vi "plot_parseDisdrometer.vi"(0 "Current Data":dbl[][](array[numeric]), 5 "Yesterday's Data":dbl[][](array[numeric])) -> (4 "Plot 1":T1(array[cluster]), 8 "Plot 2":T2(array[cluster]))   [LabVIEW 2018]
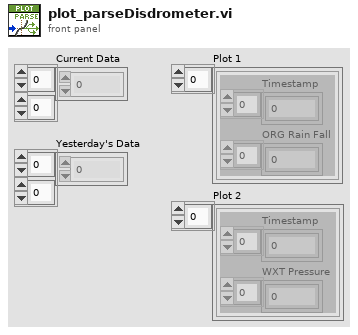
[diagram p1: front panel]
types:
  T1 = cluster{"Timestamp":dbl[], "ORG Rain Fall":dbl[]}[]
  T2 = cluster{"Timestamp":dbl[], "WXT Pressure":dbl[]}[]
  T3 = cluster{"Timestamp":dbl[], "Disdrometer Rain Rate":dbl[]}
  T4 = cluster{"Timestamp":dbl[], "Disdrometer Rain Rate":dbl[], "Disdrometer Rain Fall":dbl[]}
  T5 = cluster{"Timestamp":dbl[], "Disdrometer Rain Fall":dbl[]}
  T6 = cluster{"Timestamp":dbl[], "Disdrometer Rain Rate":dbl[]}[]
  T7 = cluster{"Timestamp":dbl[], "Disdrometer Rain Fall":dbl[]}[]
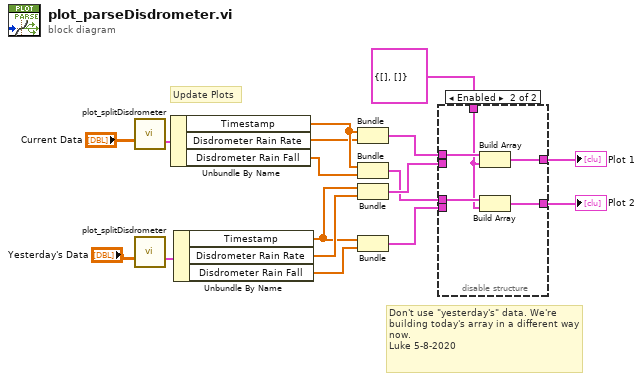
[diagram p0: block diagram]
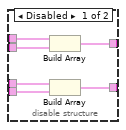
[diagram p2: hidden frame]
diagram:
  # "Don't use \"yesterday's\" data. We're building today's array in a different way now.\nLuke 5-8-2020"
  # "Update Plots"
  n1 = call "plot_splitDisdrometer.vi"("Input Arrays"="Current Data") -> ("output cluster"=w5:T4)  [unwired: 14 out]
  n2 = call "plot_splitDisdrometer.vi"("Input Arrays"="Yesterday's Data") -> ("output cluster"=w12:T4)  [unwired: 14 out]
  n3 = Unbundle By Name(w5) -> ("Timestamp"=w8:dbl[], "Disdrometer Rain Rate"=w6:dbl[], "Disdrometer Rain Fall"=w7:dbl[])
  n4 = Unbundle By Name(w12) -> ("Timestamp"=w9:dbl[], "Disdrometer Rain Rate"=w11:dbl[], "Disdrometer Rain Fall"=w10:dbl[])
  n5 = Bundle("Timestamp"=w8, "Disdrometer Rain Rate"=w6) -> (w13:T3)  [unwired: 1 out]
  n6 = Bundle("Timestamp"=w8, "Disdrometer Rain Fall"=w7) -> (w3:T5)  [unwired: 1 out]
  n7 = Bundle("Timestamp"=w9, "Disdrometer Rain Rate"=w11) -> (w14:T3)  [unwired: 1 out]
  n8 = Bundle("Timestamp"=w9, "Disdrometer Rain Fall"=w10) -> (w2:T5)  [unwired: 1 out]
  n9 = disable-structure shown="Enabled" {
    disable-tunnel: [w23 w28] -> w15
    disable-tunnel: w14 -> [w22 _]
    disable-tunnel: w13 -> [w21 w27]
    disable-tunnel: [w20 w26] -> w4
    disable-tunnel: w3 -> [w19 w25]
    disable-tunnel: w2 -> [w18 _]
    disable-tunnel: T3 {"Timestamp"=[], "Disdrometer Rain Rate"=[]} ("element") -> [_ w24]
    frame Disabled {
      n10 = Build Array(w21, w22) -> (w23:T6)
      n11 = Build Array(w19, w18) -> (w20:T7)
    }
    frame Enabled {
      n12 = Build Array(w27, w24) -> (w28:T6)
      n13 = Build Array(w25, w24) -> (w26:T6)
    }
  }
  "Plot 2" <- w4
  "Plot 1" <- w15
